vi "SVPO Envelope Detection (N Ch DBL WDT).vi"(0 "scaled signals [EU]":waveform(dbl)[](array[waveform]), 1 "reset? (F)":bool, 9 "band specification":T1={"center frequency [Hz]"=4800.0, "span [Hz]"=2000.0}) -> (4 "envelope signals [EU]":waveform(dbl)[](array[waveform]))   [LabVIEW 2017, in "SoundVib_FaultAnalysis.lvlib"]
doc: "Extracts the modulating signal, or envelope signal, from an amplitude-modulated signal. You can use the envelope detection technique to identify the mechanical faults that have amplitude-modulating effect on the vibration signal of a machine. Use this VI on embedded targets that have limited computational resources. Wire data to the <B>scaled signal [EU]</B> input to determine the polymorphic instance to use or manually select the instance."
uses:
  <vilib>/addons/Sound and Vibration/Order Analysis/Fault Analysis/SoundVib_FaultAnalysis.lvlib
  <vilib>/addons/Sound and Vibration/Order Analysis/Resample Order Tracking/SubVIs/oa_Calculate CIC Decimation Filter Coefficients.vi
  <vilib>/addons/Sound and Vibration/Order Analysis/Fault Analysis/SubVIs/sv_Compute Shift and Low Pass Filter with IC.vi
  <vilib>/addons/Sound and Vibration/Order Analysis/Resample Order Tracking/SubVIs/OAT Frequency Shift (Mixer).vi
  <vilib>/addons/Sound and Vibration/Order Analysis/Resample Order Tracking/SubVIs/oa_Decimation with CIC and Compensation Filter.vi
  <vilib>/addons/Sound and Vibration/Order Analysis/Fault Analysis/SubVIs/oa_Demodulation Initial States (1 Channel).vi
  <vilib>/addons/Sound and Vibration/Order Analysis/Adv Resampling/OAT Single Stage Decimation with IC.vi
  <vilib>/addons/Sound and Vibration/Order Analysis/Resample Order Tracking/SubVIs/OAT CIC Decimation.vi
  <vilib>/addons/Sound and Vibration/Order Analysis/Resample Order Tracking/SubVIs/oa_Interpolate Zeros Between Samples.vi
  <vilib>/addons/Sound and Vibration/Order Analysis/Resample Order Tracking/SubVIs/oa_Calculate Delay of CIC Decimation Interpolation Filter.vi
  <vilib>/addons/Sound and Vibration/Order Analysis/Resample Order Tracking/SubVIs/oa_Create CIC Compensation Filter.vi
  <vilib>/addons/Sound and Vibration/Order Analysis/Resample Order Tracking/SubVIs/oa_Create CIC LP Truncation Filter.vi
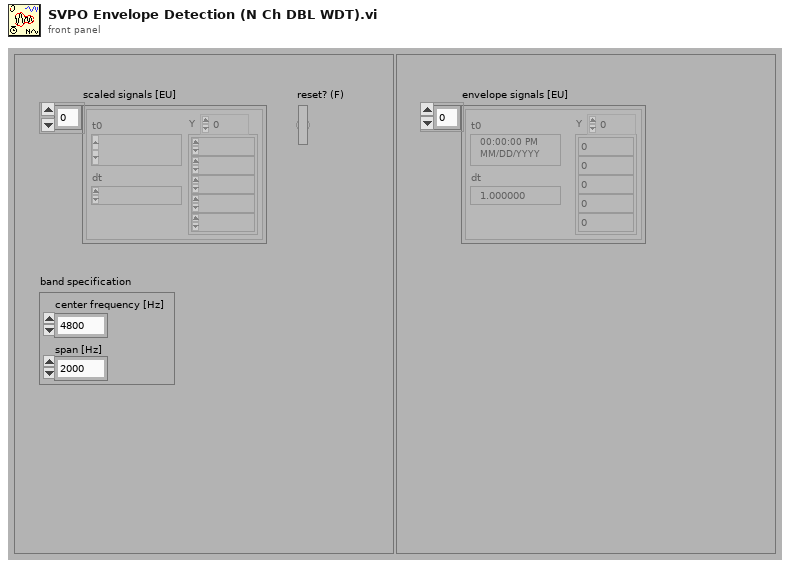
[diagram p1: front panel]
types:
  T1 = cluster{"center frequency [Hz]":dbl, "span [Hz]":dbl}
  T2 = typedef "OAT Decimation Filter.ctl" = cluster{"coefficients":dbl[], "factor":i32}
  T3 = cluster{"filter settings":cluster{"CIC Settings":cluster{"Numeric":i32, i32, i32}, "filters":T2[], "delay":i32, "interpolation factor":i32}, "filter states":cluster{"t0":dbl, "phase":dbl, "real filter state":cluster{cluster{dbl[]}, cluster{dbl[]}[]}, "imaginary filter state":cluster{cluster{dbl[]}, cluster{dbl[]}[]}, "delay":i32}[], "reset pending":bool}
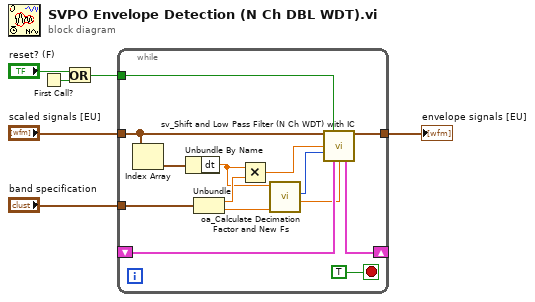
[diagram p0: block diagram]
diagram:
  n1 = First Call?() -> (First Call?: T/F=w4:bool)
  n2 = Or(x="reset? (F)", y=w4) -> (x .or. y?=w3:bool)
  n3 = while {
    tunnel: "band specification" -> [w20]
    tunnel: w3 -> [w13]
    tunnel: "scaled signals [EU]" -> [w12]
    tunnel: [w11] -> w1
    shift-right: [w9] -> _
    shift-left: _ -> [w8]
    stop <- TRUE stop-if-true
    n4 = Index Array(array=w12) -> (element=w15:waveform(dbl))  [unwired: 1 in]
    n5 = Unbundle By Name(w15) -> ("dt"=w14:dbl)
    n6 = Unbundle(w20) -> ("center frequency [Hz]"=w16:dbl, "span [Hz]"=w17:dbl)
    n7 = Multiply(x=w14, y=w16) -> (x*y=w18:dbl)
    n8 = call <vilib>:"oa_Calculate Decimation Factor and New Fs.vi"("span"=w17, "dt"=w14) -> ("new dt"=w7:dbl, "decimation factor"=w19:i32)  [unwired: 8 in]
    n9 = call <vilib>:"sv_Shift and Low Pass Filter (N Ch WDT) with IC.vi"("input signals"=w12, "reset? (F)"=w13, "center"=w18, "decimation factor"=w19, "initial conditions"=w8, "new dt"=w7) -> ("enveloped signals"=w11:waveform(dbl)[], "final conditions"=w9:T3)  [unwired: 8 in]
  }
  "envelope signals [EU]" <- w1
